vi "LED.vi"(5 "Power LED Intensity (0-255)":u8, 7 "Power LED Color (G[0]-R[255])":u8, 8 "error in":errorcluster, 9 "LEDs on":T1 items=["None"=0, "Advance"=8, "Play"=2, "Advance + Play"=10], 11 "UART port in":T2) -> (0 "error out":errorcluster, 3 "UART port out":T2)   [LabVIEW 2013]
doc: "Change the state of the iRobot power, play, and advance LEDs.\n\nThis VI writes to, but does not read from, the serial port."
uses:
  Advanced/UART/iRobot UART Port Type.ctl
  LED.ctl
  Advanced/Command/OpCode.ctl
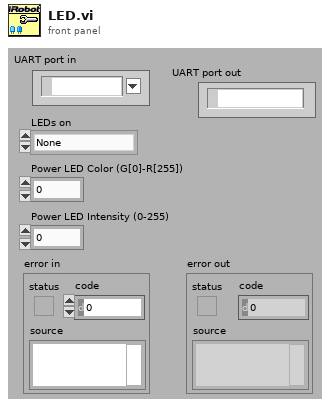
[diagram p1: front panel]
types:
  T1 = typedef "LED.ctl" = u8
  T2 = typedef "iRobot UART Port Type.ctl" = refnum<visa-resource-name>
  T3 = typedef "OpCode.ctl" = u8
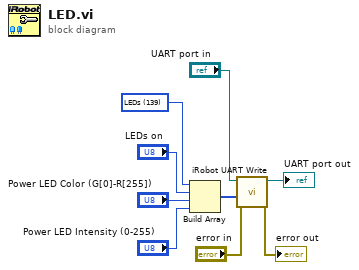
[diagram p0: block diagram]
diagram:
  w9 = T3 139 items=["Start"=128, "Baud"=129, "Control"=130, "Safe"=131, "Full"=132, "Demo"=136, "Demo - Cover"=135, "Demo - Cover and Dock"=143, "Demo - Spot"=134, "Drive"=137, "Drive Direct"=145, "LEDs"=139, "Digital Outputs"=147, "PWM Low Side Drivers"=144, "Low Side Drivers"=138, "Send IR"=151, "Song"=140, "Play Song"=141, "Sensors"=142, "Query List"=149, "Stream"=148, "Pause/Resume Stream"=150, "Script"=152, "Play Script"=153, "Show Script"=154, "Wait Time"=155, "Wait Distance"=156, "Wait Angle"=157, "Wait Event"=158] ("OpCode")
  n1 = Build Array(w9, "LEDs on", "Power LED Color (G[0]-R[255])", "Power LED Intensity (0-255)") -> (w6:T1[])
  n2 = call "iRobot UART Write.vi"("error in"="error in", "data"=w6, "UART port in"="UART port in") -> ("error out"=→"error out":errorcluster, "UART port out"=→"UART port out":T2)  [unwired: 1 in, 6 out]
